vi "Create GOODBYE msg.vi"(8 "error in":errorcluster, 11 "Termination Reason":T1) -> (0 "error out":errorcluster, 3 "String":string)   [LabVIEW 2020, in "wamplv.lvlib" / "WAMP Client.lvclass"]
uses:
  WAMP Client.lvclass
  API/TypeDefs/Termination Reason.ctl
  TypeDef/Termination Reason Enum.ctl
  TypeDef/WAMP Message Codes.ctl
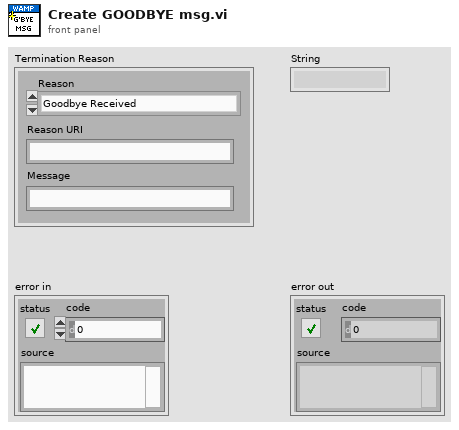
[diagram p1: front panel]
types:
  T1 = typedef "wamplv.lvlib/WAMP Client.lvclass/Termination Reason.ctl" = cluster{"Reason":T2, "Reason URI":string, "Message":string}
  T2 = typedef "wamplv.lvlib/WAMP Client.lvclass/Termination Reason Enum.ctl" = enum16{"Goodbye Received", "Abort Received", "Send Goodbye", "Send Abort", "Read Loop Failure", "Write Loop Failure", "Message Loop Failure"}
  T3 = typedef "wamplv.lvlib/WAMP Client.lvclass/WAMP Message Codes.ctl" = u16
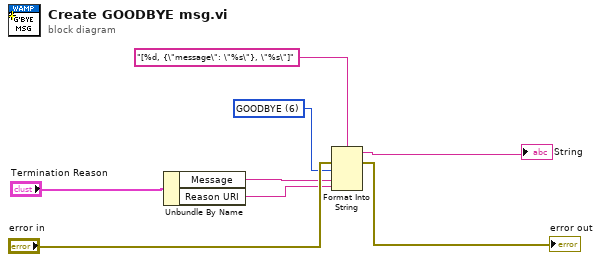
[diagram p0: block diagram]
diagram:
  w1 = T3 6 items=["HELLO"=1, "WELCOME"=2, "ABORT"=3, "GOODBYE"=6, "ERROR"=8, "PUBLISH"=16, "PUBLISHED"=17, "SUBSCRIBE"=32, "SUBSCRIBED"=33, "UNSUBSCRIBE"=34, "UNSUBSCRIBED"=35, "EVENT"=36, "CALL"=48, "RESULT"=59, "REGISTER"=64, "REGISTERED"=65, "UNREGISTER"=66, "UNREGISTERED"=67, "INVOCATION"=68, "YIELD"=70] ("Message Codes")
  n1 = Unbundle By Name("Termination Reason") -> ("Message"=w2:string, "Reason URI"=w3:string)
  n2 = Format Into String(format string="[%d, {\"message\": \"%s\"}, \"%s\"]", error in="error in", w1, w2, w3) -> (resulting string=→"String":string, error out=→"error out":errorcluster)  [unwired: 1 in]
